vi "Write Digitizer lockin channels.vi"(8 "error in (no error)":errorcluster, 10 "Digitizer lockin channels":cluster{string[]}[](array[cluster]), 11 "Lockin Digitizer Driver in":refnum<class "Lockin Digitizer Driver.lvclass">) -> (0 "error out":errorcluster, 3 "Lockin Digitizer Driver out":refnum<class "Lockin Digitizer Driver.lvclass">)   [LabVIEW 2021, in "Lockin Digitizer Driver.lvclass"]
uses:
  Lockin Digitizer Driver.lvclass
  Lockin Digitizer Driver.lvclass/Lockin Digitizer Driver.ctl
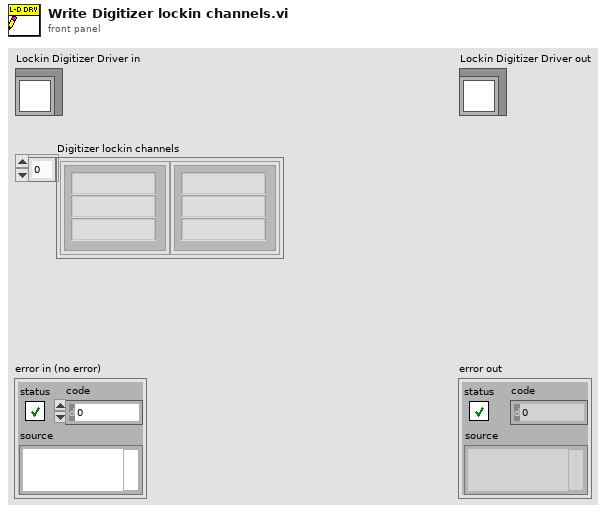
[diagram p1: front panel]
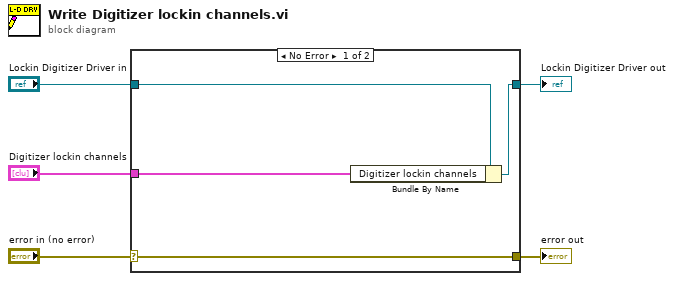
[diagram p0: block diagram]
diagram:
  n1 = case shown="No Error" "error in (no error)" {
    selector: "error in (no error)" -> [w9 w10]
    tunnel: [w9 w10] -> w4
    tunnel: [w7 w11] -> w2
    tunnel: "Lockin Digitizer Driver in" -> [w8 w11]
    tunnel: "Digitizer lockin channels" -> [w6 _]
    frame No Error {
      n2 = Bundle By Name(cluster=w8, "Digitizer lockin channels"=w6) -> (w7:refnum<class "Lockin Digitizer Driver.lvclass">)
    }
    frame Error {
    }
  }
  "error out" <- w4
  "Lockin Digitizer Driver out" <- w2
